vi "Specify component dialogue.vi"(8 "error in (no error)":errorcluster, 10 "component specification in":T2, 11 "ServiceManager in":refnum<class "ServiceManager.lvclass">) -> (0 "error out":errorcluster, 1 "path out":path, 2 "component specification out":T2, 3 "ServiceManager out":refnum<class "ServiceManager.lvclass">)   [LabVIEW 2012, in "ServiceManager.lvclass"]
uses:
  ServiceManager.lvclass
  <vilib>/Distrio/Murmex/Murmex/component_specification_cluster.ctl
  language_enum.ctl
  <vilib>/Utility/miscctls.llb/LVPointTypeDef.ctl
  <vilib>/Utility/file.llb/Read From Spreadsheet File (string).vi
  <vilib>/Distrio/Murmex/Murmex/Murmex.lvclass
panel:
  in  "button:component_search":bool
  in  "Component":string
  in  "Language":T1
  in  "button:cancel":bool
  in  "button:ok":bool
  in  "button:randomString":bool
  in  "ID":string
  in  "button:localHost":bool
  in  "Host name":string
  # "Specify a component"
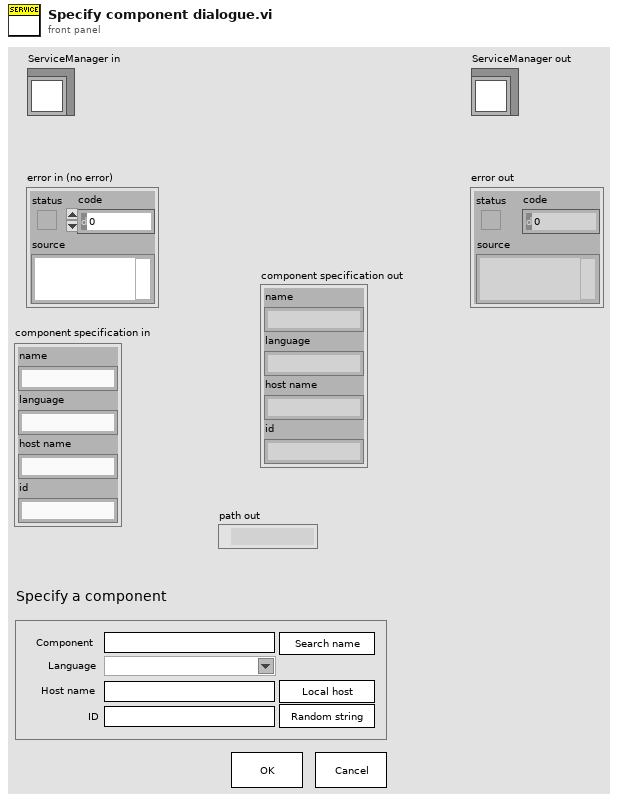
[diagram p1: front panel]
types:
  T1 = typedef "ServiceManager.lvclass/language_enum.ctl" = string
  T2 = typedef "Murmex.lvlib/Murmex.lvclass/component_specification_cluster.ctl" = cluster{"name":string, "language":string, "host name":string, "id":string}
  T3 = typedef "LVPointTypeDef.ctl" = cluster{"Horizontal":i16, "Vertical":i16}
  T4 = enum16{"open", "replace", "create", "open or create", "replace or create", "replace or create with confirmation"}
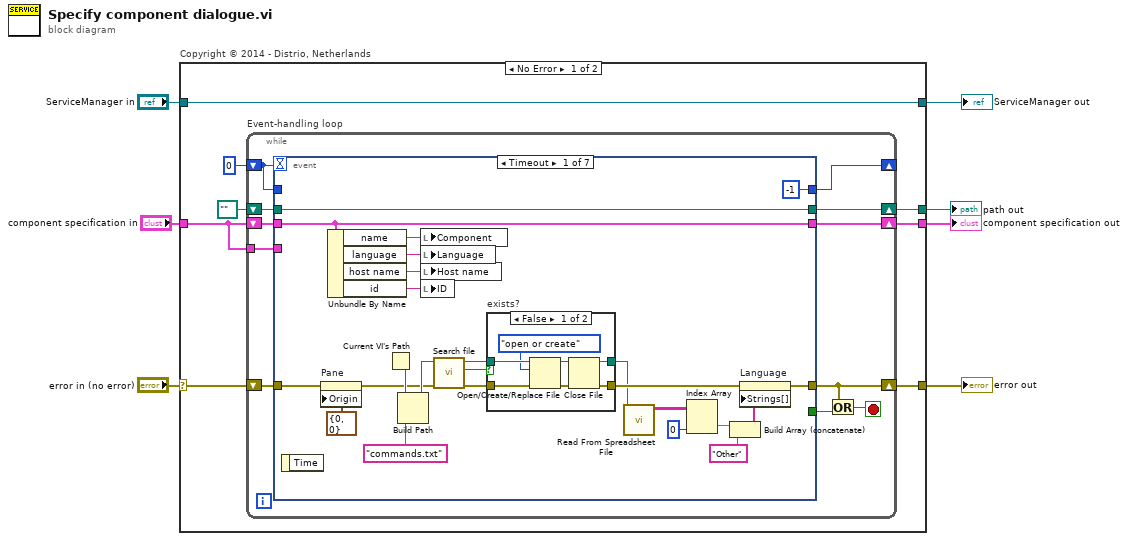
[diagram p0: block diagram]
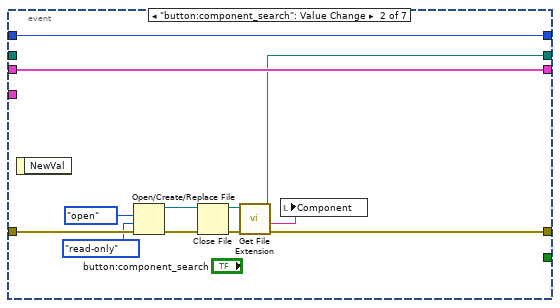
[diagram p3: hidden frame]
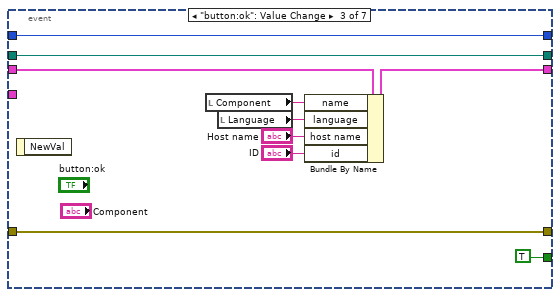
[diagram p4: hidden frame]
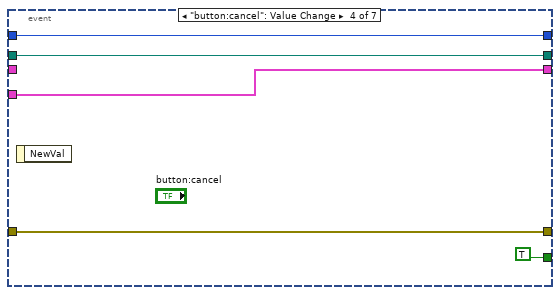
[diagram p5: hidden frame]
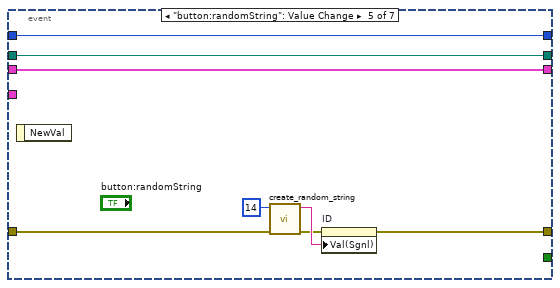
[diagram p6: hidden frame]
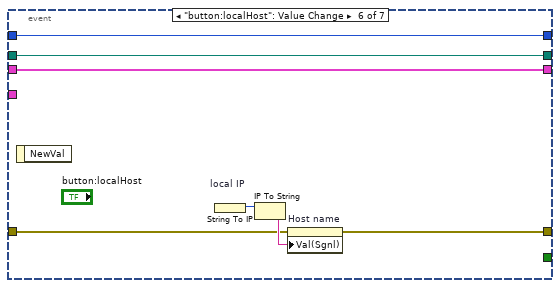
[diagram p7: hidden frame]
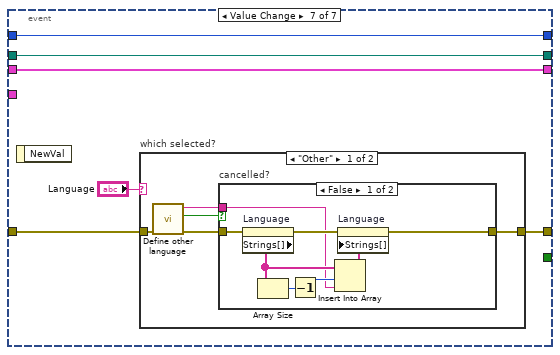
[diagram p8: hidden frame]
diagram:
  n1 = case "Copyright © 2014 - Distrio, Netherlands" shown="No Error" "error in (no error)" {
    selector: "error in (no error)" -> [w9 w125]
    tunnel: [w15 w125] -> w6
    tunnel: [w13 w124] -> w4
    tunnel: "ServiceManager in" -> [w13 w124]
    tunnel: "component specification in" -> [w8 w123]
    tunnel: [w12 w123] -> w2
    tunnel: [w11 _] -> w1
    frame No Error {
      n2 = while "Event-handling loop" {
        shift-right: [w25] -> w15
        shift-left: w9 -> [w26]
        shift-right: [w21] -> w12
        shift-left: w8 -> [w22]
        tunnel: w8 -> [w20]
        shift-right: [w18] -> _
        shift-left: 0 -> [w19]
        shift-right: [w17] -> w11
        shift-left: path "" ("dup file") -> [w16]
        stop <- w24 stop-if-true
        n3 = event shown="[0] Timeout" {
          selector: _ -> [_ _ _ _ _ _ _]
          dyn-events: _ -> [_ _ _ _ _ _ _]
          timeout: w19 -> [_ _ _ _ _ _ _]
          tunnel: w26 -> [w35 w65 w81 w86 w90 w99 w103]
          tunnel: [w38 w68 w81 w86 w94 w98 w104] -> w25
          tunnel: [_ _ TRUE TRUE _ _ _] -> w23
          tunnel: w22 -> [w45 w71 w75 _ w93 w97 w107]
          tunnel: [w45 w71 w74 w83 w93 w97 w107] -> w21
          tunnel: w20 -> [_ _ _ w83 _ _ _]
          tunnel: [-1 w70 w79 w84 w88 w96 w106] -> w18
          tunnel: w19 -> [_ w70 w79 w84 w88 w96 w106]
          tunnel: [w37 w62 w72 w82 w87 w95 w102] -> w17
          tunnel: w16 -> [w37 _ w72 w82 w87 w95 w102]
          event Timeout {
            n4 = event-data() -> ()  [unwired: 1 in, 1 out]
            n5 = property on="Pane" class="Pane"(error in=w35, "Origin"=T3 {"Horizontal"=0, "Vertical"=0}) -> (error out=w28:errorcluster)  [unwired: 1 in, 1 out]
            n6 = Unbundle By Name(w45) -> ("name"=w46:string, "language"=w49:string, "host name"=w48:string, "id"=w47:string)
            n7 = Current VI's Path() -> (path=w29:path)
            n8 = Build Path(base path=w29, name or relative path="commands.txt") -> (appended path=w31:path)
            n9 = local write "Component"(w46) -> ()
            n10 = local write "Language"(w49) -> ()
            n11 = local write "Host name"(w48) -> ()
            n12 = local write "ID"(w47) -> ()
            n13 = call <vilib>:"Search file.vi"("error in (no error)"=w28, "path in"=w31) -> ("error out"=w27:errorcluster, "found?"=w32:bool, "path out"=w30:path)  [unwired: 7 in]
            n14 = case "exists?" shown="False" w32 {
              tunnel: w27 -> [w56 w58]
              tunnel: w30 -> [w57 w59]
              tunnel: [w53 w59] -> w33
              tunnel: [w52 w58] -> w34
              frame False {
                n15 = Open/Create/Replace File(file path (use dialog)=w57, error in=w56, operation (0:open)=T4."open or create") -> (refnum out=w54:refnum<file>, error out=w55:errorcluster)  [unwired: 3 in, 1 out]
                n16 = Close File(refnum=w54, error in=w55) -> (path=w53:path, error out=w52:errorcluster)
              }
              frame True {
              }
            }
            n17 = call-poly <vilib>:"Read From Spreadsheet File.vi"("file path (dialog if empty)"=w33) -> ("all rows"=w43:string[][])  [unwired: 6 in, 4 out]
            n18 = Index Array(array=w43, index (col)=0 ("disabled index (col)")) -> (element=w41:string[])  [unwired: 1 in]
            n19 = Build Array (concatenate)(w41, "Other" ("name or relative path")) -> (w39:string[])
            n20 = property on="Language" class="CmbBox (strict)"(error in=w34, "Strings[]"=w39) -> (error out=w38:errorcluster)  [unwired: 1 in, 1 out]
          }
          event "button:component_search": Value Change {
            n21 = event-data() -> ()  [unwired: 1 in, 1 out]
            n22 = Open/Create/Replace File(error in=w65, operation (0:open)=T4."open", access (0:read/write)=enum16{"read/write", "read-only", "write-only"}."read-only") -> (refnum out=w64:refnum<file>, error out=w67:errorcluster)  [unwired: 3 in, 1 out]
            n23 = Close File(refnum=w64, error in=w67) -> (path=w63:path, error out=w66:errorcluster)
            n24 = call <vilib>:"Get File Extension.vi"("error in (no error)"=w66, "file"=w63) -> ("error out"=w68:errorcluster, "filename without extension"=w69:string, "dup file"=w62:path)  [unwired: 6 in, 1 out]
            n25 = local write "Component"(w69) -> ()
          }
          event "button:ok": Value Change {
            n26 = event-data() -> ()  [unwired: 1 in, 1 out]
            n27 = local read "Component"() -> (w76:string)
            n28 = local read "Language"() -> (w73:T1)
            n29 = Bundle By Name(cluster=w75, "name"=w76, "language"=w73, "host name"="Host name", "id"="ID") -> (w74:T2)
          }
          event "button:cancel": Value Change {
            n30 = event-data() -> ()  [unwired: 1 in, 1 out]
          }
          event "button:randomString": Value Change {
            n31 = event-data() -> ()  [unwired: 1 in, 1 out]
            n32 = call <vilib>:"create_random_string.vi"("error in (no error)"=w90, "length"=14) -> ("error out"=w89:errorcluster, "random string"=w92:string)  [unwired: 8 in]
            n33 = property on="ID" class="Str"(error in=w89, "Val(Sgnl)"=w92) -> (error out=w94:errorcluster)  [unwired: 1 in, 1 out]
          }
          event "button:localHost": Value Change {
            n34 = event-data() -> ()  [unwired: 1 in, 1 out]
            n35 = String To IP "local IP"() -> (0:w101:u32)  [unwired: 1 in]
            n36 = IP To String(2:w101) -> (0:w100:string)  [unwired: 1 in]
            n37 = property on="Host name" class="Str"(error in=w99, "Val(Sgnl)"=w100) -> (error out=w98:errorcluster)  [unwired: 1 in, 1 out]
          }
          event Value Change {
            n38 = event-data() -> ()  [unwired: 1 in, 1 out]
            n39 = case "which selected?" shown="\"Other\"" "Language" {
              tunnel: [w110 w122] -> w104
              tunnel: w103 -> [w112 w122]
              frame "Other" {
                n40 = call "Define other language.vi"("error in (no error)"=w112) -> ("error out"=w109:errorcluster, "cancelled?"=w111:bool, "language out"=w108:string)  [unwired: 8 in]
                n41 = case "cancelled?" shown="False" w111 {
                  tunnel: [w118 w121] -> w110
                  tunnel: w109 -> [w120 w121]
                  tunnel: w108 -> [w113 _]
                  frame False {
                    n42 = property on="Language" class="CmbBox (strict)"(error in=w120) -> (error out=w119:errorcluster, "Strings[]"=w117:string[])  [unwired: 1 in, 1 out]
                    n43 = Array Size(array=w117) -> (size(s)=w115:i32)
                    n44 = Decrement(x=w115) -> (x-1=w116:i32)
                    n45 = Insert Into Array(array=w117, index=w116, new element=w113) -> (w114:string[])
                    n46 = property on="Language" class="CmbBox (strict)"(error in=w119, "Strings[]"=w114) -> (error out=w118:errorcluster)  [unwired: 1 in, 1 out]
                  }
                  frame True {
                  }
                }
              }
              frame Default {
              }
            }
          }
        }
        n47 = Or(x=w25, y=w23) -> (x .or. y?=w24:bool)
      }
    }
    frame Error {
    }
  }
  "error out" <- w6
  "ServiceManager out" <- w4
  "component specification out" <- w2
  "path out" <- w1
